vi "Delete Resource.vi"(6 "Remote Timeout (300,000 ms)":u32=300000, 8 "error in (no error)":errorcluster, 10 "Delete Mode":i32(ring) items=["validate but do not delete"=-1, "delete if no dependencies exist"=0, "delete item and any dependencies"=1, "delete item but keep dependencies"=2], 11 "Resource in":refnum<k20>) -> (0 "error out":errorcluster, 2 "Detailed Result":string, 3 "Resource out":refnum<k20>, 4 "Dependent Items Deleted":bool)   [LabVIEW 2020, in "nisyscfg.lvlib"]
doc: "Permanently removes a hardware resource and its configuration data from the system. Not all devices can be deleted; consult your product documentation."
uses:
  <vilib>/nisyscfg/nisyscfg.lvlib
  <vilib>/Utility/error.llb/Error Cluster From Error Code.vi
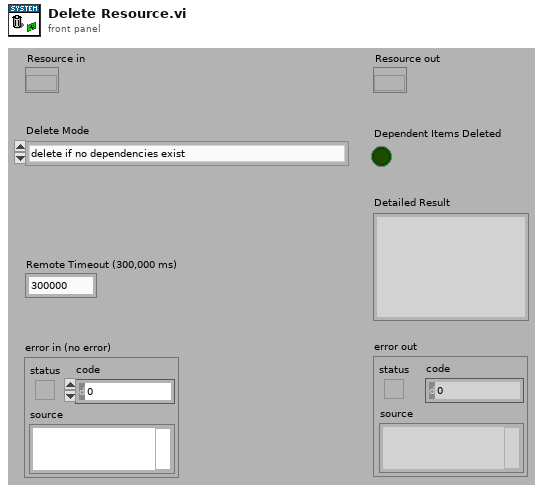
[diagram p1: front panel]
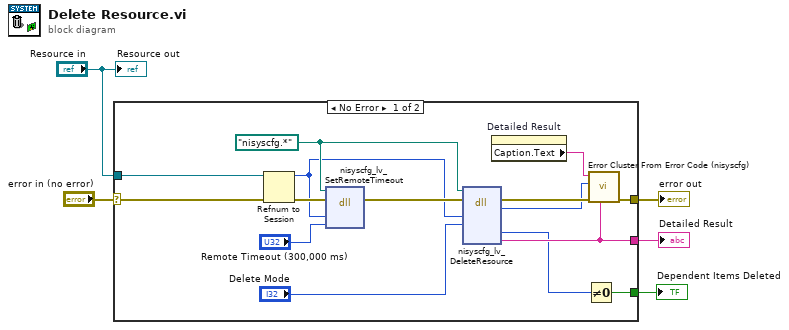
[diagram p0: block diagram]
diagram:
  n1 = case shown="No Error" "error in (no error)" {
    selector: "error in (no error)" -> [w13 w21]
    tunnel: [w18 w21] -> w5
    tunnel: "Resource in" -> [w10 _]
    tunnel: [w17 _] -> w2
    tunnel: [w6 _] -> w1
    frame No Error {
      w11 = path "nisyscfg.*" ("path in")
      n2 = Refnum to Session(4:w13, 7:w10) -> (0:w14:errorcluster, 3:w9:u64)
      n3 = dll-call lib="nisyscfg.*" fn="nisyscfg_lv_SetRemoteTimeout" label="SetRemoteTimeout"(path in=w11, error in=w14, "item"=w9, "connectTimeout"="Remote Timeout (300,000 ms)") -> (error out=w12:errorcluster)  [unwired: 1 in, 4 out]
      n4 = dll-call lib="nisyscfg.*" fn="nisyscfg_lv_DeleteResource" label="DeleteResource"(path in=w11, error in=w12, "itemToDelete"=w9, "deleteMode"="Delete Mode") -> (error out=w19:errorcluster, "return type"=w15:i32, "moreDeleted"=w7:u8, "detailedResult"=w17:string)  [unwired: 5 in, 1 out]
      n5 = property on="Detailed Result" class="Str"() -> ("Caption.Text"=w16:string)  [unwired: 2 in, 2 out]
      n6 = Not Equal To 0?(x=w7) -> (x != 0?=w6:bool)
      n7 = call <vilib>:"Error Cluster From Error Code (nisyscfg).vi"("Details String"=w17, "error in (no error)"=w19, "Error Code (0)"=w15, "Details Caption"=w16) -> ("error out"=w18:errorcluster)  [unwired: 7 in]
    }
    frame Error {
    }
  }
  "error out" <- w5
  "Detailed Result" <- w2
  "Dependent Items Deleted" <- w1
  "Resource out" <- "Resource in"
